vi "subCheckPathAndName.vi"(4 "exclude instances?":bool, 6 "parent path":path, 10 "delimited name":string, 11 "path":path) -> (2 "path out":path, 3 "path to check?":bool)   [LabVIEW 2020, in "DependencyInspection.lvlib" / "CDependencyInspection.lvclass"]
uses:
  CDependencyInspection.lvclass
  CommonHelpers/CommonHelpers.lvlib
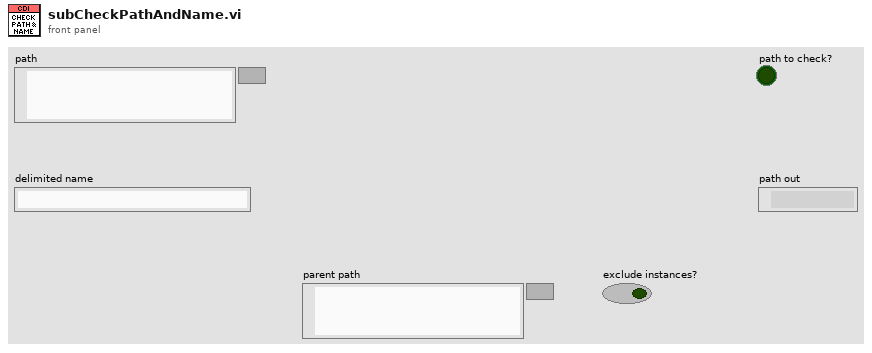
[diagram p1: front panel]
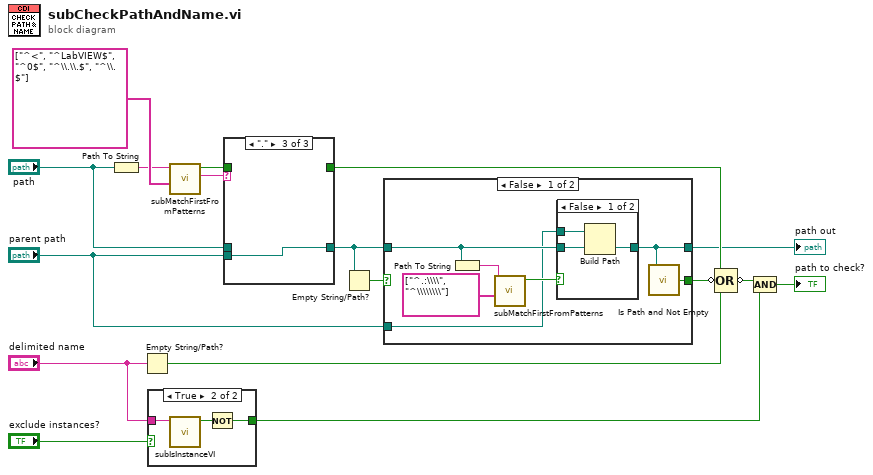
[diagram p0: block diagram]
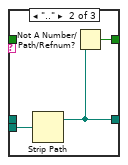
[diagram p5: hidden frame]
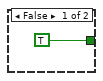
[diagram p6: hidden frame]
diagram:
  n1 = Path To String(path="path") -> (string=w8:string)
  n2 = Empty String/Path?(string/path="delimited name") -> (empty?=w17:bool)
  n3 = case shown="True" "exclude instances?" {
    tunnel: [TRUE w19] -> w16
    tunnel: "delimited name" -> [_ w20]
    frame False {
    }
    frame True {
      n4 = call "subIsInstanceVI.vi"("delimited name"=w20) -> ("found?"=w21:bool)  [unwired: 10 in]
      n5 = Not(x=w21) -> (.not. x?=w19:bool)
    }
  }
  n6 = call "subMatchFirstFromPatterns.vi"("patterns"=string[] ["^<", "^LabVIEW$", "^0$", "^\\.\\.$", "^\\.$"], "string in"=w8) -> ("matched string"=w11:string, "found?"=w9:bool)  [unwired: 7 in, 1 out]
  n7 = case shown="\".\"" w11 {
    tunnel: [w23 w25 _] -> w10
    tunnel: w9 -> [w23 _ _]
    tunnel: "parent path" -> [_ w26 w27]
    tunnel: "path" -> [w22 _ _]
    tunnel: [w22 w24 w27] -> w3
    frame Default {
    }
    frame ".." {
      n8 = Strip Path(path=w26) -> (stripped path=w24:path)  [unwired: 1 out]
      n9 = Not A Number/Path/Refnum?(number/path/refnum=w24) -> (NaN/Path/Refnum?=w25:bool)
    }
    frame "." {
    }
  }
  n10 = Empty String/Path?(string/path=w3) -> (empty?=w6:bool)
  n11 = case shown="False" w6 {
    selector: w6 -> [_ w40]
    tunnel: [w29 w40] -> w5
    tunnel: [w30 w39] -> w4
    tunnel: w3 -> [w31 w39]
    tunnel: "parent path" -> [w28 _]
    frame False {
      n12 = Path To String(path=w31) -> (string=w34:string)
      n13 = call "subMatchFirstFromPatterns.vi"("patterns"=string[] ["^.:\\\\", "^\\\\\\\\"], "string in"=w34) -> ("found?"=w32:bool)  [unwired: 7 in, 2 out]
      n14 = case shown="False" w32 {
        tunnel: w31 -> [w36 w38]
        tunnel: w28 -> [w37 _]
        tunnel: [w35 w38] -> w30
        frame False {
          n15 = Build Path(base path=w37, name or relative path=w36) -> (appended path=w35:path)
        }
        frame True {
        }
      }
      n16 = call <vilib>:"Is Path and Not Empty.vi"("path"=w30) -> ("Is Path and Not Empty?"=w29:bool)  [unwired: 4 in]
    }
    frame True {
    }
  }
  "path out" <- w4
  n17 = Compound Arithmetic op=OR(w10, invert w5, w17) -> (invert w1:bool)
  n18 = Compound Arithmetic op=AND(w1, w16) -> (→"path to check?":bool)
